vi "Build Major Frame Start.vi"(7 "Virtual Memory Unit in":refnum<class "Virtual Memory Unit.lvclass">, 8 "error in (no error)":errorcluster, 10 "Starting Address":u16 format="%04x", 11 "Major Frame in":refnum<class "Major Frame.lvclass">) -> (0 "error out":errorcluster, 2 "Next Available Address":u16 format="%04x", 3 "Major Frame out":refnum<class "Major Frame.lvclass">, 5 "Virtual Memory Unit out":refnum<class "Virtual Memory Unit.lvclass">)   [LabVIEW 2020, in "BCI-1553 API.lvlib" / "Major Frame.lvclass"]
doc: "The first few commands of the Major Frame will be to load up the minor frame timer and start it. Additionally, we track the input address as the first address used for the instruction list. This address will be the formal 'start address' for all further instruction list operations."
uses:
  Major Frame.lvclass
  Dependencies/Virtual Memory Unit/Virtual Memory Unit.lvclass
  TypeDefs/BC Op Codes - Verbose.ctl
  TypeDefs/BC Condition Codes.ctl
  Major Frame.lvclass/Major Frame.ctl
  BCI-1553 API.lvlib
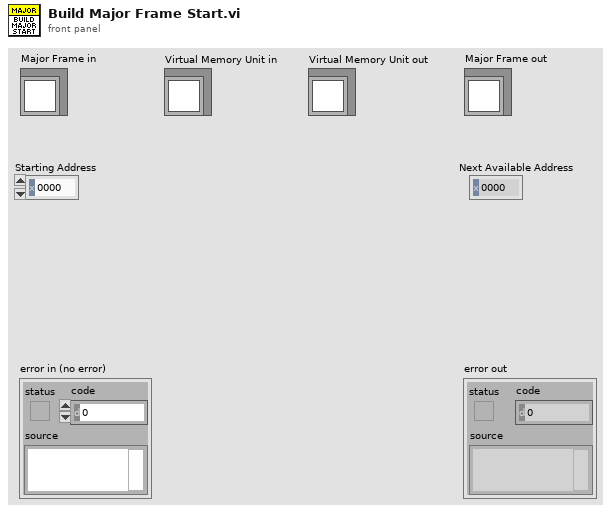
[diagram p1: front panel]
types:
  T1 = typedef "BCI-1553 API.lvlib/BC Op Codes - Verbose.ctl" = enum16{"EXECUTE MSG", "EXECUTE MSG GO", "JUMP", "CALL SUBROUTINE", "RETURN", "INTERRUPT REQUEST", "HALT", "DELAY", "WAIT FRAME TIMER = 0", "COMPARE FRAME TIMER", "COMPARE MSG TIMER", "LOAD TIME TAG CTR", "LOAD TIME TAG CTR HI", "LOAD FRAME TIMER", "START FRAME TIMER", "PUSH TIME TAG COUNT", "PUSH TIME TAG COUNT HI", "PUSH TIME TAG COUNT BOTH", "PUSH BLOCK STATUS WORD", "PUSH CURRENT VALUE", "PUSH INDIRECT", "WAIT EXT TRIGGER", "EXECUTE AND FLIP", "EXECUTE, FLIP, GO", "WRITE VALUE TO WMI", "WRITE VALUE TO MEM", "DECREMENT RAM, SKIP", "FLAG"}
  T2 = typedef "BCI-1553 API.lvlib/BC Condition Codes.ctl" = enum16{"GP0 == 1 || LT", "GP1 == 1 || NE", "GP2 == 1", "GP3 == 1", "GP4 == 1", "GP5 == 1", "GP6 == 1", "GP7 == 1", "NORESP", "FMTERR", "GOODBLOCK", "MSKSTATSET", "BADMSG", "1RETRY", "2RETRY", "ALWAYS"}
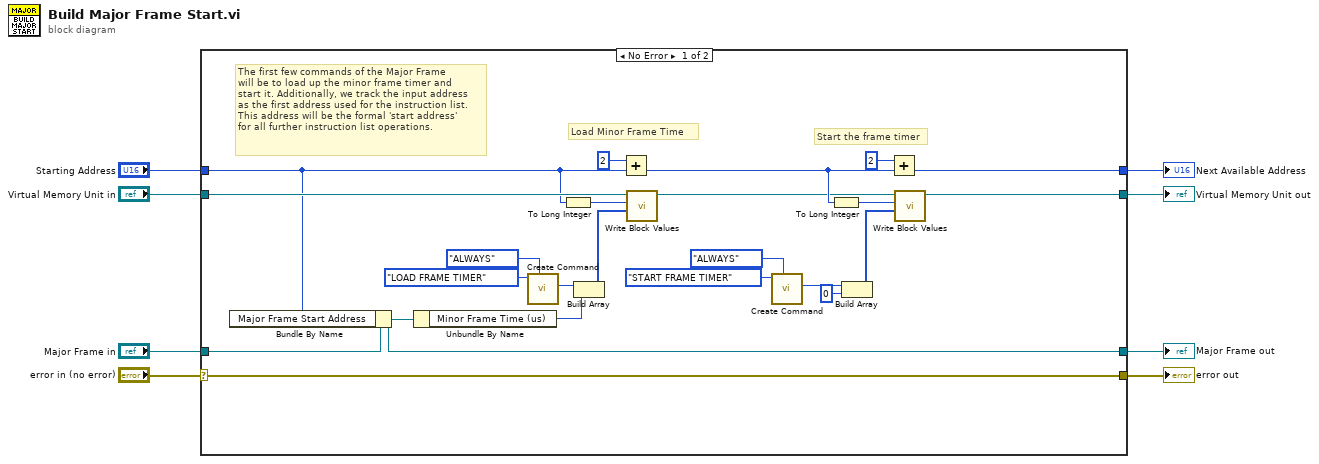
[diagram p0: block diagram]
diagram:
  n1 = case shown="No Error" "error in (no error)" {
    selector: "error in (no error)" -> [w31 w35]
    tunnel: [w31 w35] -> w7
    tunnel: [w29 w34] -> w5
    tunnel: "Major Frame in" -> [w30 w34]
    tunnel: [w9 w32] -> w4
    tunnel: "Virtual Memory Unit in" -> [w27 w32]
    tunnel: [w12 w33] -> w2
    tunnel: "Starting Address" -> [w22 w33]
    frame No Error {
      # "Start the frame timer"
      # "Load Minor Frame Time"
      # "The first few commands of the Major Frame\nwill be to load up the minor frame timer and\nstart it. Additionally, we track the input address\nas the first address used for the instruction list.\nThis address will be the formal 'start address'\nfor all further instruction list operations."
      n2 = Bundle By Name(cluster=w30, "Major Frame Start Address"=w22) -> (w29:refnum<class "Major Frame.lvclass">)
      n3 = Unbundle By Name(w29) -> ("Minor Frame Time (us)"=w25:u16)
      n4 = call "Create Command.vi"("Condition"=BC_Condition_Codes."ALWAYS", "Op Code"=BC_Op_Codes_-_Verbose."LOAD FRAME TIMER") -> ("Instruction"=w24:u16)  [unwired: 8 in, 1 out]
      n5 = To Long Integer(number=w22) -> (32bit integer=w21:i32)
      n6 = Build Array(w24, w25) -> (w20:u16[])
      n7 = Add(x=u16 2, y=w22) -> (x+y=w13:u16)
      n8 = call "Write Block Values.vi"("Write Block"=w20, "Start Index"=w21, "Virtual Memory Unit in"=w27) -> ("Virtual Memory Unit out"=w10:refnum<class "Virtual Memory Unit.lvclass">)  [unwired: 7 in, 1 out]
      n9 = call "Create Command.vi"("Condition"=BC_Condition_Codes."ALWAYS", "Op Code"=BC_Op_Codes_-_Verbose."START FRAME TIMER") -> ("Instruction"=w16:u16)  [unwired: 8 in, 1 out]
      n10 = To Long Integer(number=w13) -> (32bit integer=w18:i32)
      n11 = Build Array(w16, u16 0 ("element")) -> (w19:u16[])
      n12 = Add(x=u16 2, y=w13) -> (x+y=w12:u16)
      n13 = call "Write Block Values.vi"("Write Block"=w19, "Start Index"=w18, "Virtual Memory Unit in"=w10) -> ("Virtual Memory Unit out"=w9:refnum<class "Virtual Memory Unit.lvclass">)  [unwired: 7 in, 1 out]
    }
    frame Error {
    }
  }
  "error out" <- w7
  "Major Frame out" <- w5
  "Virtual Memory Unit out" <- w4
  "Next Available Address" <- w2
